vi "Update Method Accessor.vi"(6 "accessor type":T1="Get", 7 "library":refnum<vi>, 8 "error in (no error)":errorcluster, 9 "method message metadata name":string, 10 "rpc method name":string, 11 "server class in":refnum<vi>) -> (0 "error out":errorcluster, 3 "server class out":refnum<vi>)   [LabVIEW 2019, in "gRPC Template Creation Utility.lvlib"]
uses:
  gRPC Template Creation Utility.lvlib
  TypeDefs/Method Accessor Type.ctl
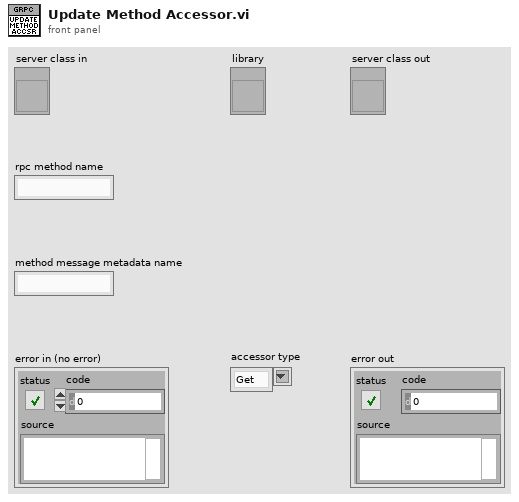
[diagram p1: front panel]
types:
  T1 = typedef "gRPC Template Creation Utility.lvlib/Method Accessor Type.ctl" = string
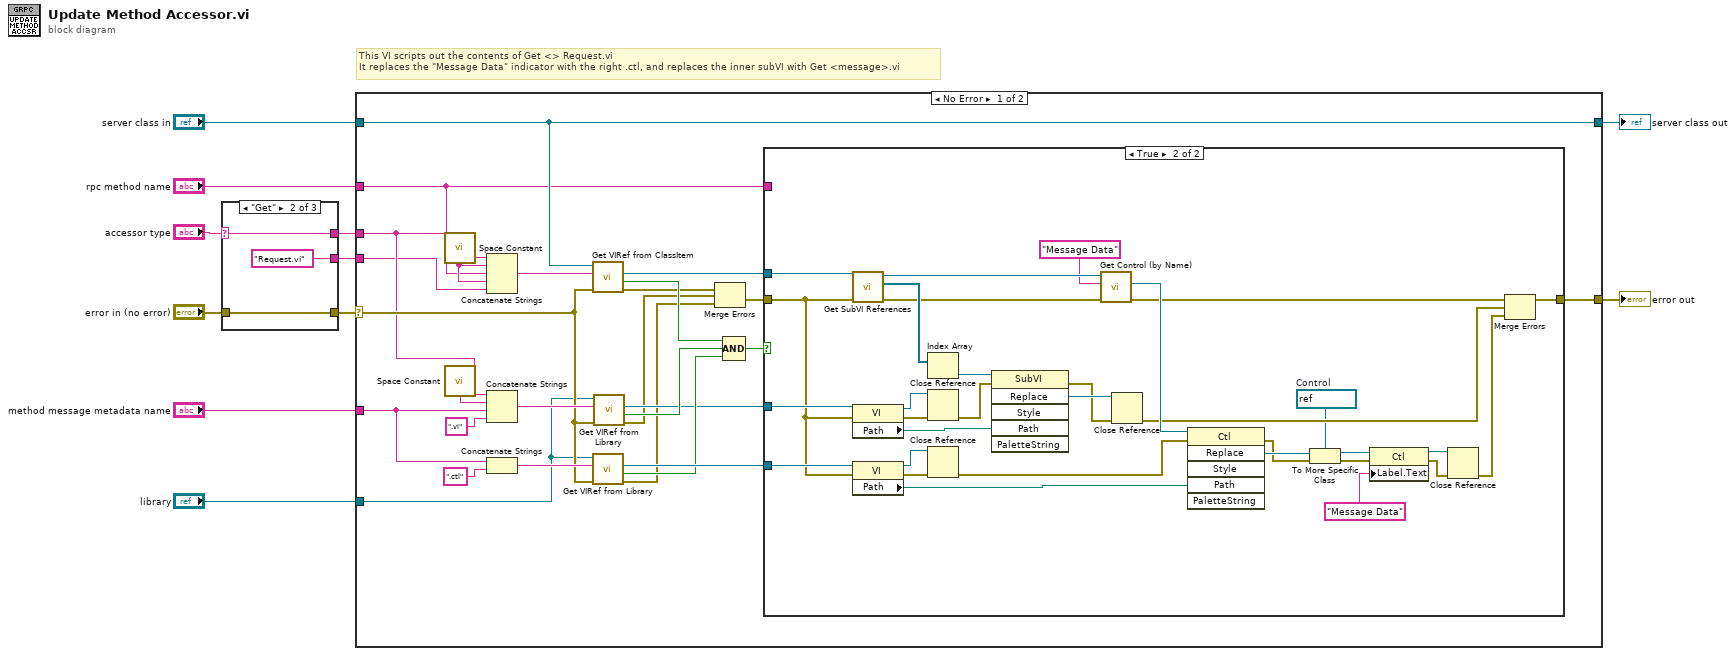
[diagram p0: block diagram]
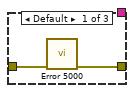
[diagram p2: hidden frame]
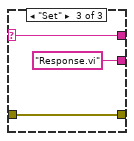
[diagram p3: hidden frame]
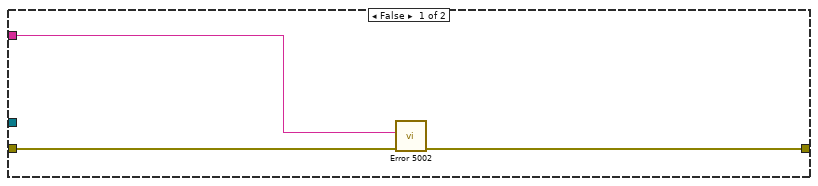
[diagram p4: hidden frame]
diagram:
  # "This VI scripts out the contents of Get <> Request.vi\nIt replaces the \"Message Data\" indicator with the right .ctl, and replaces the inner subVI with Get <message>.vi"
  n1 = case shown="\"Get\"" "accessor type" {
    selector: "accessor type" -> [_ w16 w19]
    tunnel: [_ w16 w19] -> w2
    tunnel: [_ "Request.vi" ("string") "Response.vi" ("string")] -> w1
    tunnel: "error in (no error)" -> [w13 w14 w17]
    tunnel: [w12 w14 w17] -> w3
    frame Default {
      n2 = call "Error 5000.vi"("error in (no error)"=w13) -> ("error out"=w12:errorcluster)  [unwired: 10 in]
    }
    frame "Get" {
    }
    frame "Set" {
    }
  }
  n3 = case shown="No Error" w3 {
    selector: w3 -> [w30 w82]
    tunnel: "server class in" -> [w24 w81]
    tunnel: "method message metadata name" -> [w38 _]
    tunnel: "rpc method name" -> [w23 _]
    tunnel: [w25 w82] -> w8
    tunnel: [w24 w81] -> w7
    tunnel: "library" -> [w22 _]
    tunnel: w2 -> [w21 _]
    tunnel: w1 -> [w20 _]
    frame No Error {
      n4 = call <vilib>:"Space Constant.vi"() -> ("String"=w31:string)
      n5 = call <vilib>:"Space Constant.vi"() -> ("String"=w32:string)
      n6 = Concatenate Strings(w21, w31, w23, w31, w20) -> (w35:string)
      n7 = Concatenate Strings(w21, w32, w38, ".vi" ("string")) -> (w34:string)
      n8 = Concatenate Strings(w38, ".ctl" ("string")) -> (w40:string)
      n9 = call "Get VIRef from ClassItem.vi"("error in (no error)"=w30, "Item Name"=w35, "LVClassLibrary in"=w24) -> ("error out"=w29:errorcluster, "Found ?"=w41:bool, "VIref out"=w36:refnum<vi>)  [unwired: 5 in, 1 out]
      n10 = call "Get VIRef from Library.vi"("error in (no error)"=w30, "Item Name"=w40, "Library"=w22) -> ("error out"=w26:errorcluster, "Found ?"=w43:bool, "VIref out"=w45:refnum<vi>)  [unwired: 5 in, 1 out]
      n11 = call "Get VIRef from Library.vi"("error in (no error)"=w30, "Item Name"=w34, "Library"=w22) -> ("error out"=w27:errorcluster, "Found ?"=w42:bool, "VIref out"=w37:refnum<vi>)  [unwired: 5 in, 1 out]
      n12 = Merge Errors(w29, w27, w26) -> (w28:errorcluster)
      n13 = Compound Arithmetic op=AND(w41, w42, w43) -> (w44:bool)
      n14 = case shown="True" w44 {
        tunnel: w36 -> [_ w78]
        tunnel: w37 -> [_ w77]
        tunnel: w45 -> [_ w73]
        tunnel: w28 -> [w48 w67]
        tunnel: [w47 w49] -> w25
        tunnel: w23 -> [w46 _]
        frame False {
          n15 = call "Error 5002.vi"("error in (no error)"=w48, "Method Name"=w46) -> ("error out"=w47:errorcluster)  [unwired: 9 in]
        }
        frame True {
          w56 = refnum<vi> refnum  # Control
          n16 = call "Get SubVI References.vi"("error in (no error)"=w67, "Owner vi in"=w78) -> ("error out"=w68:errorcluster, "SubVI refs"=w80:refnum<vi>[], "Owner vi out"=w71:refnum<vi>)  [unwired: 7 in]
          n17 = property class="VI"(reference=w77, error in=w67) -> (reference out=w63:refnum<vi>, error out=w64:errorcluster, "Path"=w76:path)
          n18 = property class="VI"(reference=w73, error in=w67) -> (reference out=w61:refnum<vi>, error out=w62:errorcluster, "Path"=w72:path)
          n19 = Index Array(array=w80) -> (element=w79:refnum<vi>)  [unwired: 1 in]
          n20 = Close Reference(reference=w63, error in (no error)=w64) -> (error out=w59:errorcluster)
          n21 = Close Reference(reference=w61, error in (no error)=w62) -> (error out=w60:errorcluster)
          n22 = invoke class="SubVI" method="Replace"(reference=w79, error in=w59, "Path"=w76) -> (error out=w74:errorcluster, "Replace"=w75:refnum<vi>)  [unwired: 3 in, 4 out]
          n23 = call "Get Control (by Name).vi"("error in (no error)"=w68, "Control Label"="Message Data" ("Constant Label"), "Owner VI in"=w71) -> ("error out"=w66:errorcluster, "Control Refnum"=w69:refnum<vi>)  [unwired: 5 in, 2 out]
          n24 = Close Reference(reference=w75, error in (no error)=w74) -> (error out=w65:errorcluster)
          n25 = invoke class="Ctl" method="Replace"(reference=w69, error in=w60, "Path"=w72) -> (error out=w57:errorcluster, "Replace"=w58:refnum<vi>)  [unwired: 3 in, 4 out]
          n26 = To More Specific Class(target class=w56, reference=w58, error in=w57) -> (specific class reference=w54:refnum<vi>, error out=w55:errorcluster)
          n27 = property class="Ctl"(reference=w54, error in=w55, "Label.Text"="Message Data") -> (reference out=w51:refnum<vi>, error out=w52:errorcluster)
          n28 = Close Reference(reference=w51, error in (no error)=w52) -> (error out=w50:errorcluster)
          n29 = Merge Errors(w66, w65, w50) -> (w49:errorcluster)
        }
      }
    }
    frame Error {
    }
  }
  "server class out" <- w7
  "error out" <- w8
